vi "Radix.vi"(8 "error in (no error)":errorcluster, 10 "radix":enum8{"hide", "dec", "hex", "bin"}(ring), 11 "GObject in":refnum<vi>) -> (0 "error out":errorcluster, 2 "has radix?":bool, 3 "GObject out":refnum<vi>)   [LabVIEW 2019, in "Builtins.lvlib"]
doc: "Changes the numeric or string radix on the selected front panel or block diagram object. \n\nOption: Numeric == String\ndec: Decimal '0d' == Normal Text 'n'\nhex: Hex '0x' == Hexadecimal Text 'x'\nbin: Binary '0b' == Backslash Text '\\'\nhide: Hide Radix\n\nCreated by: Ryan Pacini"
uses:
  Builtins.lvlib
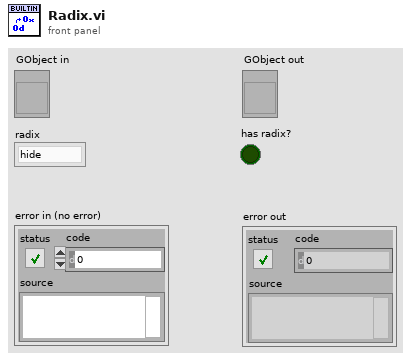
[diagram p1: front panel]
types:
  T1 = typedef "LVNumericRepresentation.ctl" = enum32{"Extended Precision", "Double Precision", "Single Precision", "Long", "Word", "Byte", "Unsigned Long", "Unsigned Word", "Unsigned Byte", "Complex Extended", "Complex Double", "Complex Single", "Quad", "Unsigned Quad", "Fixed-Point"}
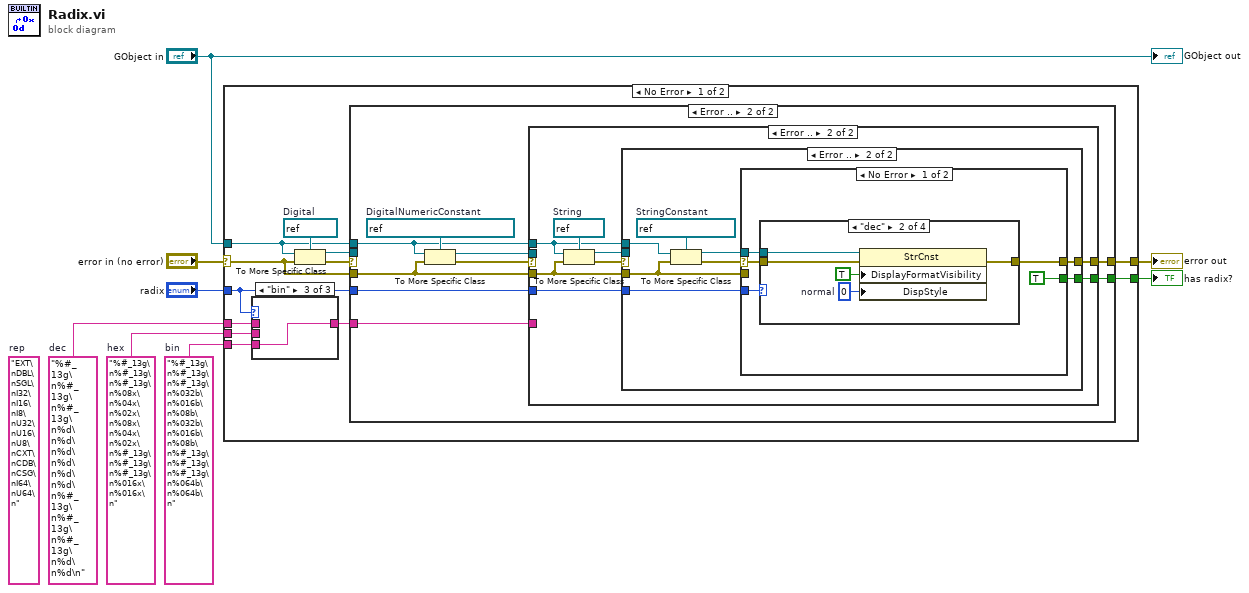
[diagram p0: block diagram]
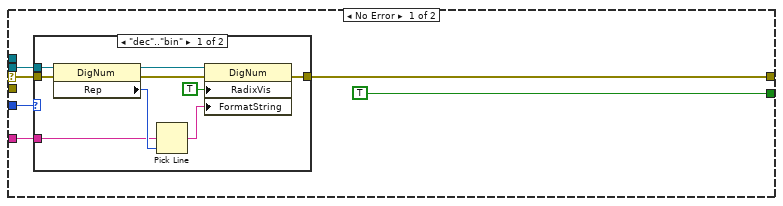
[diagram p4: hidden frame]
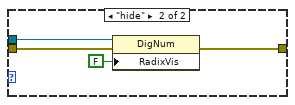
[diagram p5: hidden frame]
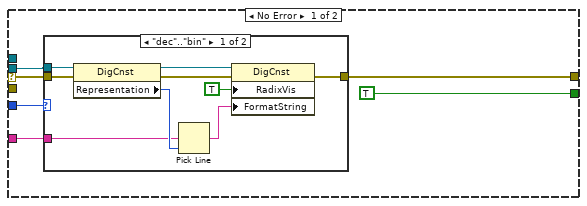
[diagram p6: hidden frame]
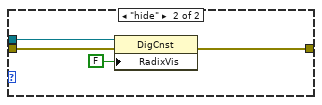
[diagram p7: hidden frame]
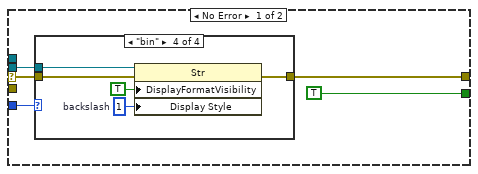
[diagram p8: hidden frame]
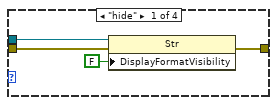
[diagram p9: hidden frame]
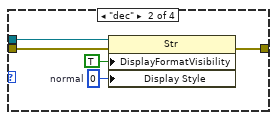
[diagram p10: hidden frame]
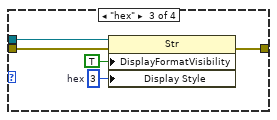
[diagram p11: hidden frame]
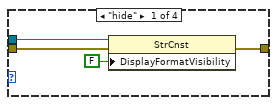
[diagram p12: hidden frame]
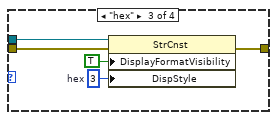
[diagram p13: hidden frame]
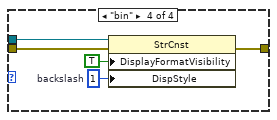
[diagram p14: hidden frame]
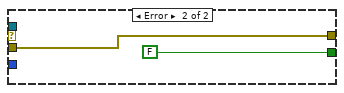
[diagram p15: hidden frame]
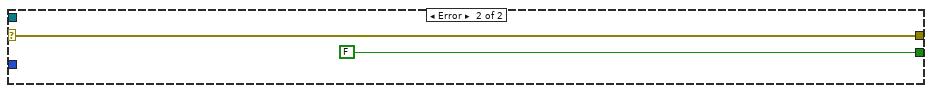
[diagram p16: hidden frame]
diagram:
  (unwired) "EXT\nDBL\nSGL\nI32\nI16\nI8\nU32\nU16\nU8\nCXT\nCDB\nCSG\nI64\nU64\n"  # rep
  w1 = "%#_13g\n%#_13g\n%#_13g\n%032b\n%016b\n%08b\n%032b\n%016b\n%08b\n%#_13g\n%#_13g\n%#_13g\n%064b\n%064b\n"  # bin
  w2 = "%#_13g\n%#_13g\n%#_13g\n%08x\n%04x\n%02x\n%08x\n%04x\n%02x\n%#_13g\n%#_13g\n%#_13g\n%016x\n%016x\n"  # hex
  w3 = "%#_13g\n%#_13g\n%#_13g\n%d\n%d\n%d\n%d\n%d\n%d\n%#_13g\n%#_13g\n%#_13g\n%d\n%d\n"  # dec
  n1 = case shown="No Error" "error in (no error)" {
    selector: "error in (no error)" -> [w16 w138]
    tunnel: "GObject in" -> [w18 _]
    tunnel: "radix" -> [w14 _]
    tunnel: [w20 w138] -> w6
    tunnel: [w15 FALSE] -> w5
    tunnel: w3 -> [w13 _]
    tunnel: w2 -> [w12 _]
    tunnel: w1 -> [w11 _]
    frame No Error {
      w19 = refnum<vi> refnum  # Digital
      n2 = case shown="\"bin\"" w14 {
        tunnel: w13 -> [w21 _ _]
        tunnel: w12 -> [_ w22 _]
        tunnel: w11 -> [_ _ w23]
        tunnel: [w21 w22 w23] -> w10
        frame "hide", "dec" {
        }
        frame "hex" {
        }
        frame "bin" {
        }
      }
      n3 = To More Specific Class(target class=w19, reference=w18, error in=w16) -> (specific class reference=w9:refnum<vi>, error out=w17:errorcluster)
      n4 = case shown="Error .." w17 {
        selector: w17 -> [w24 _]
        tunnel: w14 -> [w28 w47]
        tunnel: [w26 w48] -> w20
        tunnel: w18 -> [_ w44]
        tunnel: w16 -> [_ w45]
        tunnel: [TRUE w43] -> w15
        tunnel: w10 -> [w27 w46]
        tunnel: w9 -> [w25 _]
        frame No Error {
          n5 = case shown="\"dec\"..\"bin\"" w28 {
            tunnel: w24 -> [w36 w41]
            tunnel: w25 -> [w34 w40]
            tunnel: [w37 w42] -> w26
            tunnel: w27 -> [w31 _]
            frame "dec".."bin" {
              n6 = property class="DigNum"(reference=w34, error in=w36) -> (reference out=w33:refnum<vi>, error out=w35:errorcluster, "Rep"=w32:T1)
              n7 = Pick Line(multi-line string=w31, line index=w32) -> (output string=w30:string)  [unwired: 1 in]
              n8 = property class="DigNum"(reference=w33, error in=w35, "RadixVis"=TRUE ("Radix Visible?"), "FormatString"=w30) -> (error out=w37:errorcluster)  [unwired: 1 out]
            }
            frame "hide" {
              n9 = property class="DigNum"(reference=w40, error in=w41, "RadixVis"=FALSE ("Radix Visible?")) -> (error out=w42:errorcluster)  [unwired: 1 out]
            }
          }
        }
        frame Error {
          w51 = refnum<vi> refnum  # DigitalNumericConstant
          n10 = To More Specific Class(target class=w51, reference=w44, error in=w45) -> (specific class reference=w49:refnum<vi>, error out=w50:errorcluster)
          n11 = case shown="Error .." w50 {
            selector: w50 -> [w57 _]
            tunnel: w49 -> [w56 _]
            tunnel: [w55 w74] -> w48
            tunnel: w47 -> [w54 w75]
            tunnel: w46 -> [w53 _]
            tunnel: w45 -> [_ w73]
            tunnel: w44 -> [_ w72]
            tunnel: [TRUE w71] -> w43
            frame No Error {
              n12 = case shown="\"dec\"..\"bin\"" w54 {
                tunnel: w57 -> [w64 w69]
                tunnel: w56 -> [w62 w68]
                tunnel: [w65 w70] -> w55
                tunnel: w53 -> [w59 _]
                frame "dec".."bin" {
                  n13 = property class="DigCnst"(reference=w62, error in=w64) -> (reference out=w61:refnum<vi>, error out=w63:errorcluster, "Representation"=w60:T1)
                  n14 = Pick Line(multi-line string=w59, line index=w60) -> (output string=w58:string)  [unwired: 1 in]
                  n15 = property class="DigCnst"(reference=w61, error in=w63, "RadixVis"=TRUE ("Radix Visible?"), "FormatString"=w58) -> (error out=w65:errorcluster)  [unwired: 1 out]
                }
                frame "hide" {
                  n16 = property class="DigCnst"(reference=w68, error in=w69, "RadixVis"=FALSE ("Radix Visible?")) -> (error out=w70:errorcluster)  [unwired: 1 out]
                }
              }
            }
            frame Error {
              w78 = refnum<vi> refnum  # String
              n17 = To More Specific Class(target class=w78, reference=w72, error in=w73) -> (specific class reference=w76:refnum<vi>, error out=w77:errorcluster)
              n18 = case shown="Error .." w77 {
                selector: w77 -> [w83 _]
                tunnel: w76 -> [w82 _]
                tunnel: w75 -> [w81 w106]
                tunnel: [w80 w105] -> w74
                tunnel: w73 -> [_ w104]
                tunnel: w72 -> [_ w109]
                tunnel: [TRUE w103] -> w71
                frame No Error {
                  n19 = case shown="\"bin\"" w81 {
                    tunnel: w83 -> [w86 w91 w96 w101]
                    tunnel: w82 -> [w85 w90 w95 w100]
                    tunnel: [w87 w92 w97 w102] -> w80
                    frame "hide" {
                      n20 = property class="Str"(reference=w85, error in=w86, "DisplayFormatVisibility"=FALSE ("Display Format Visible?")) -> (error out=w87:errorcluster)  [unwired: 1 out]
                    }
                    frame "dec" {
                      w88 = u32 0  # normal
                      n21 = property class="Str"(reference=w90, error in=w91, "DisplayFormatVisibility"=TRUE ("Display Format Visible?"), "Display Style"=w88) -> (error out=w92:errorcluster)  [unwired: 1 out]
                    }
                    frame "hex" {
                      w93 = u32 3  # hex
                      n22 = property class="Str"(reference=w95, error in=w96, "DisplayFormatVisibility"=TRUE ("Display Format Visible?"), "Display Style"=w93) -> (error out=w97:errorcluster)  [unwired: 1 out]
                    }
                    frame "bin" {
                      w98 = u32 1  # backslash
                      n23 = property class="Str"(reference=w100, error in=w101, "DisplayFormatVisibility"=TRUE ("Display Format Visible?"), "Display Style"=w98) -> (error out=w102:errorcluster)  [unwired: 1 out]
                    }
                  }
                }
                frame Error {
                  w110 = refnum<vi> refnum  # StringConstant
                  n24 = To More Specific Class(target class=w110, reference=w109, error in=w104) -> (specific class reference=w107:refnum<vi>, error out=w108:errorcluster)
                  n25 = case shown="No Error" w108 {
                    selector: w108 -> [w115 _]
                    tunnel: w107 -> [w114 _]
                    tunnel: w106 -> [w113 _]
                    tunnel: [w112 w136] -> w105
                    tunnel: w104 -> [_ w136]
                    tunnel: [TRUE FALSE] -> w103
                    frame No Error {
                      n26 = case shown="\"dec\"" w113 {
                        tunnel: w115 -> [w118 w123 w128 w133]
                        tunnel: w114 -> [w117 w122 w127 w132]
                        tunnel: [w119 w124 w129 w134] -> w112
                        frame "hide" {
                          n27 = property class="StrCnst"(reference=w117, error in=w118, "DisplayFormatVisibility"=FALSE ("Display Format Visible?")) -> (error out=w119:errorcluster)  [unwired: 1 out]
                        }
                        frame "dec" {
                          w120 = u32 0  # normal
                          n28 = property class="StrCnst"(reference=w122, error in=w123, "DisplayFormatVisibility"=TRUE ("Display Format Visible?"), "DispStyle"=w120) -> (error out=w124:errorcluster)  [unwired: 1 out]
                        }
                        frame "hex" {
                          w125 = u32 3  # hex
                          n29 = property class="StrCnst"(reference=w127, error in=w128, "DisplayFormatVisibility"=TRUE ("Display Format Visible?"), "DispStyle"=w125) -> (error out=w129:errorcluster)  [unwired: 1 out]
                        }
                        frame "bin" {
                          w130 = u32 1  # backslash
                          n30 = property class="StrCnst"(reference=w132, error in=w133, "DisplayFormatVisibility"=TRUE ("Display Format Visible?"), "DispStyle"=w130) -> (error out=w134:errorcluster)  [unwired: 1 out]
                        }
                      }
                    }
                    frame Error {
                    }
                  }
                }
              }
            }
          }
        }
      }
    }
    frame Error {
    }
  }
  "error out" <- w6
  "has radix?" <- w5
  "GObject out" <- "GObject in"
